vi "Random Aberration Array Generator.vi"(9 "max random order":i64, 10 "aberration tolerance":dbl format="%#_13g", 11 "aberration threshold":dbl format="%#_13g") -> (2 "Zer coeff":dbl[](array[numeric]), 3 "Zer index (starting from 3)":dbl[](array[numeric]))   [LabVIEW 2018]
uses:
  <vilib>/Analysis/1siggen.llb/Ramp Pattern by Delta.vi
  <vilib>/Analysis/NI_AALBase.lvlib
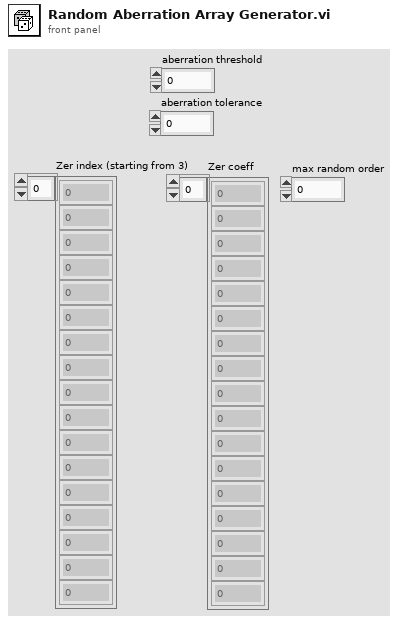
[diagram p1: front panel]
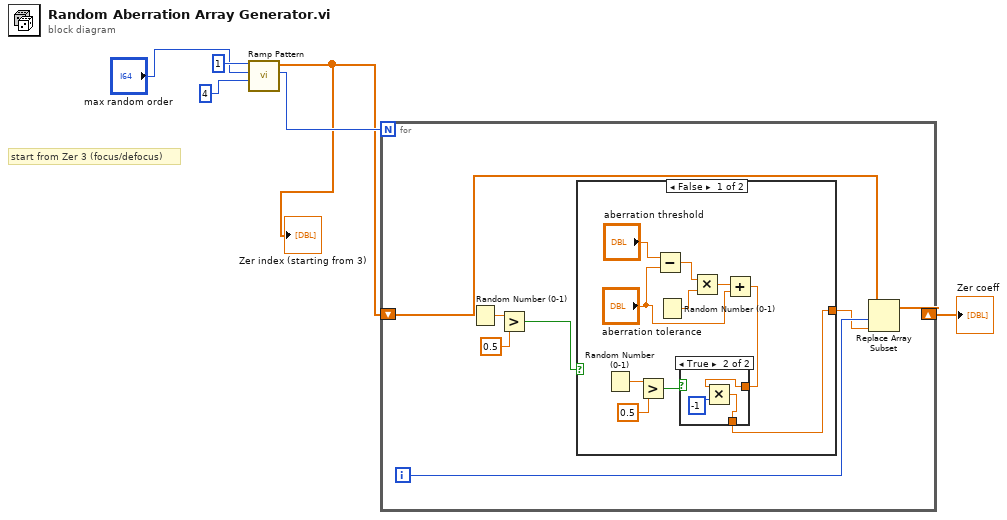
[diagram p0: block diagram]
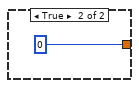
[diagram p3: hidden frame]
diagram:
  # "start from Zer 3 (focus/defocus)"
  n1 = call-poly <vilib>:"Ramp Pattern.vi"("start"=4, "end"="max random order", "delta"=1) -> ("samples"=w3:i32, "Ramp Pattern"=w1:dbl[])  [unwired: 6 in, 1 out]
  "Zer index (starting from 3)" <- w1
  n2 = for {
    N: w3 -> [_]
    shift-right: [w12] -> w2
    shift-left: w1 -> [w11]
    i -> [w13]
    n3 = Random Number (0-1)() -> (number: 0 to 1=w10:dbl)
    n4 = Greater?(x=w10, y=0.5) -> (0:w8:bool)
    n5 = case shown="False" w8 {
      tunnel: [w14 0] -> w7
      frame False {
        n6 = Random Number (0-1)() -> (number: 0 to 1=w18:dbl)
        n7 = Greater?(x=w18, y=0.5) -> (0:w16:bool)
        n8 = Subtract(x="aberration threshold", y="aberration tolerance") -> (x-y=w22:dbl)
        n9 = Random Number (0-1)() -> (number: 0 to 1=w21:dbl)
        n10 = Multiply(x=w22, y=w21) -> (x*y=w20:dbl)
        n11 = Add(x=w20, y="aberration tolerance") -> (x+y=w15:dbl)
        n12 = case shown="True" w16 {
          tunnel: w15 -> [w24 w25]
          tunnel: [w24 w27] -> w14
          frame False {
          }
          frame True {
            n13 = Multiply(x=w25, y=-1) -> (x*y=w27:dbl)
          }
        }
      }
      frame True {
      }
    }
    n14 = Replace Array Subset(array=w11, new element=w7, index=w13) -> (w12:dbl[])
  }
  "Zer coeff" <- w2
